vi "Keithley6221Monitor_with_DC.vi"() -> ()   [LabVIEW 2019]
uses:
  Instrument_Setup.vi
  Global/Global Variables/Data_Display_global.vi
  <vilib>/ErrorRing/Error Ring.xnode
  Equipment/Keithley 622x/Keithley 622x.lvlib
  Utility/Monitor Communication/sub-vis/K6221_Check_Queue.vi
  Utility/Monitor Communication/sub-vis/K6221_Open_Queue.vi
  Utility/Monitor Communication/K6221/K6221_Cluster.ctl
  Equipment/Keithley 622x/Configure/Output/Typedefs/KE6221 -- Output Response.ctl
  Equipment/Keithley 622x/Typedefs/KE622x -- On Off Control.ctl
  Equipment/Keithley 622x/Configure/Source/Typedefs/KE622x -- Voltage Limit.ctl
  Equipment/Keithley 622x/Configure/Source/Typedefs/KE622x -- Current Ranges.ctl
  Equipment/Keithley 622x/Configure/Source/Typedefs/KE622x -- Current Range.ctl
panel:
  in  "Current Range In":T1={"Auto Range?"=TRUE, "Man / Selected\nRange"=enum."2nA"}
  in  "Turn Off Output If Voltage Limit? 2":bool=TRUE
  in  "Turn Off Output If Voltage Limit?":bool=TRUE
  in  "Voltage Limit (V)":T3=10.0 min=0.1 max=105.0 step=0.01 format="%.2p"
  in  "Analog Filter State":T4
  in  "Output Response":T5=enum."Slow"
  in  "Combo Box":string(combo)="AC"
  out "Cluster":T6
  # "Set in Instrument Setup!"
  # "K 6221"
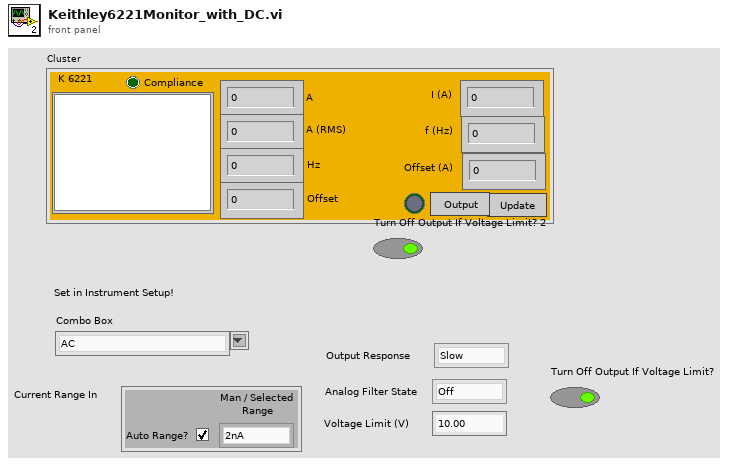
[diagram p1: front panel]
types:
  T1 = typedef "Keithley 622x.lvlib/KE622x -- Current Range.ctl" = cluster{"Auto Range?":bool, "Man / Selected\nRange":T2}
  T2 = typedef "Keithley 622x.lvlib/KE622x -- Current Ranges.ctl" = enum16{"2nA", "20nA", "200nA", "2uA", "20uA", "200uA", "2mA", "20mA", "100mA"}
  T3 = typedef "Keithley 622x.lvlib/KE622x -- Voltage Limit.ctl" = dbl
  T4 = typedef "Keithley 622x.lvlib/KE622x -- On Off Control.ctl" = enum16{"Off", "On"}
  T5 = typedef "Keithley 622x.lvlib/KE6221 -- Output Response.ctl" = enum16{"Fast", "Slow"}
  T6 = typedef "K6221_Cluster.ctl" = cluster{"Plot Window":dbl[][], "A":dbl, "A (RMS)":dbl, "Hz":dbl, "I (A)":dbl, "f (Hz)":dbl, "Update":bool, "Offset":dbl, "Offset (A)":dbl, "Compliance":bool, "Output":bool, "Output Status":bool}
  T7 = typedef "Keithley 622x.lvlib/KE622x -- Current Level.ctl" = dbl
  T8 = typedef "Keithley 622x.lvlib/KE6221 -- Wave Sine Wave Params.ctl" = cluster{"Frequency (Hz)":T9, "Amplitude (A)":T10, "Offset (A)":T7, "Ranging Mode":T11, "Fixed Range":T2, "Playback Mode":T12, "Time (s)":T13, "Num Cycles":T14, "Phase\nMarker?":bool, "Phase Marker (deg)":T15, "Trig Link Line":T16}
  T9 = typedef "Keithley 622x.lvlib/KE6221 -- Wave Frequency.ctl" = dbl
  T10 = typedef "Keithley 622x.lvlib/KE6221 -- Wave Amplitude.ctl" = dbl
  T11 = typedef "Keithley 622x.lvlib/KE6221 -- Wave Ranging Mode.ctl" = enum16{"Best", "Fixed"}
  T12 = typedef "Keithley 622x.lvlib/KE6221 -- Wave Playback Mode.ctl" = enum16{"Time", "Num Cycles"}
  T13 = typedef "Keithley 622x.lvlib/KE6221 -- Wave Playback Time.ctl" = dbl
  T14 = typedef "Keithley 622x.lvlib/KE6221 -- Wave Playback Num Cycles.ctl" = dbl
  T15 = typedef "Keithley 622x.lvlib/KE6221 -- Wave Phase Marker.ctl" = dbl
  T16 = typedef "Keithley 622x.lvlib/KE622x -- Trig Link Line.ctl" = enum16{"1", "2", "3", "4", "5", "6"}
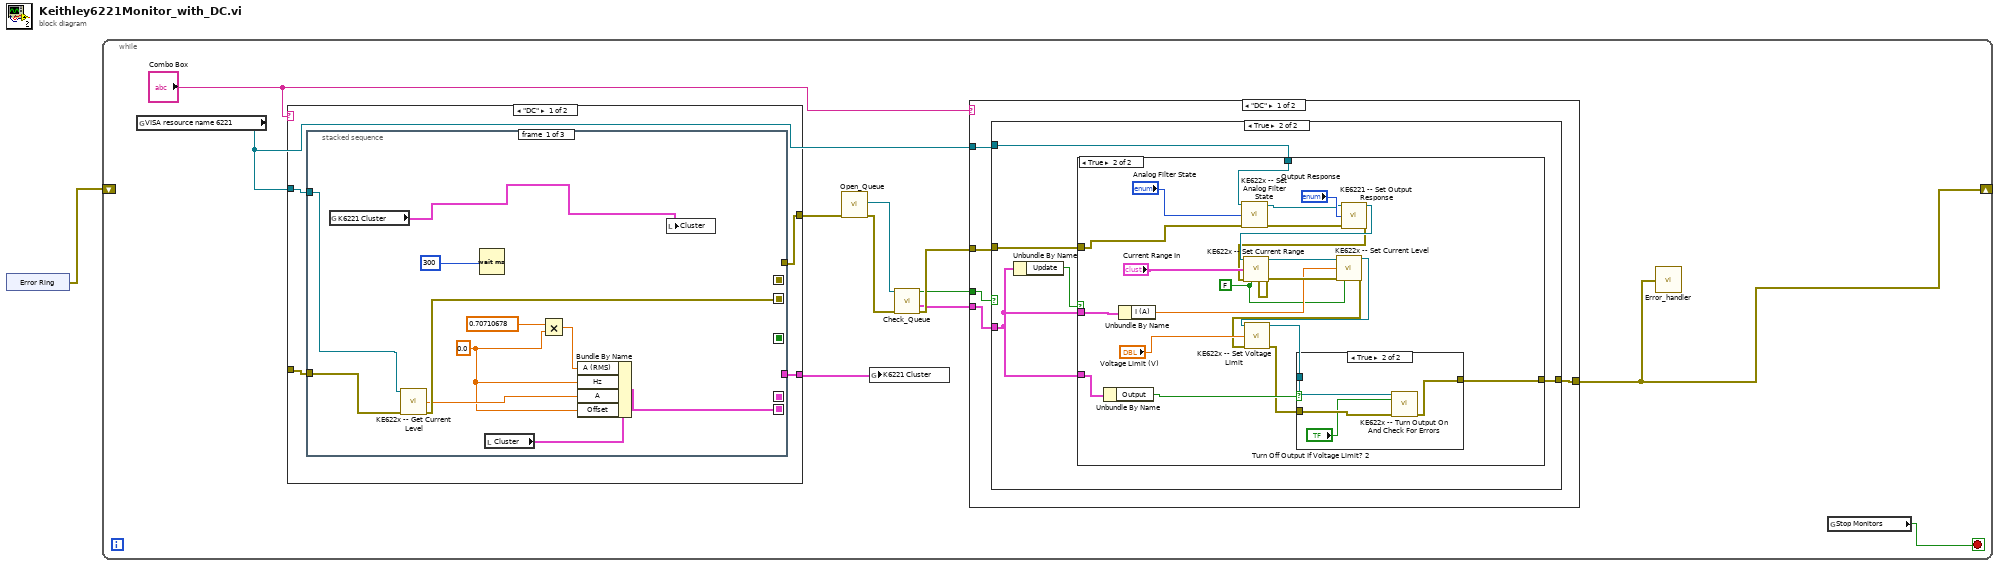
[diagram p0: block diagram]
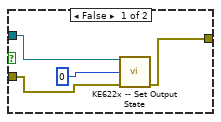
[diagram p4: hidden frame]
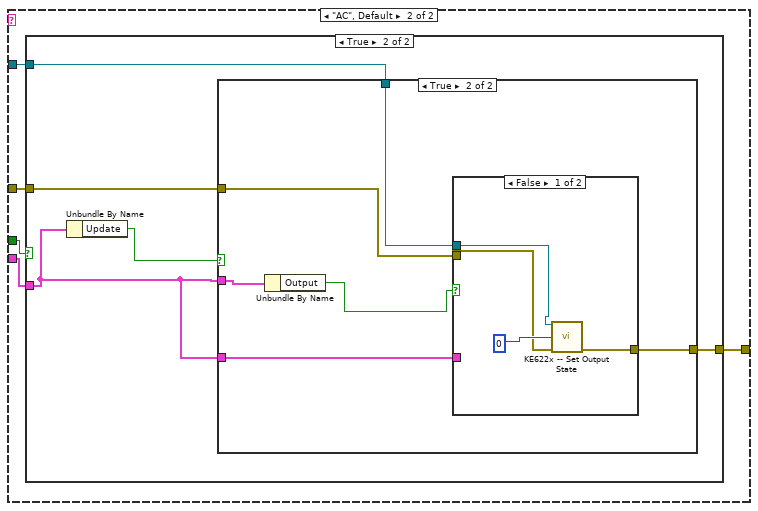
[diagram p5: hidden frame]
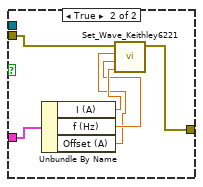
[diagram p8: hidden frame]
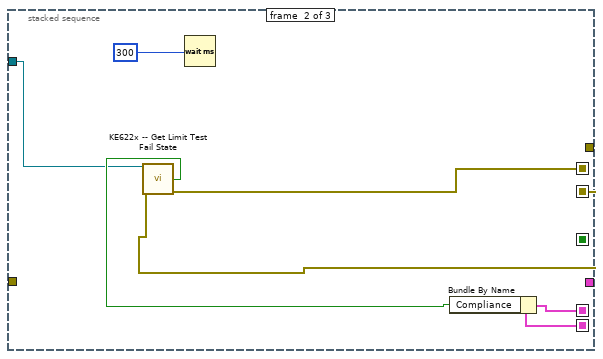
[diagram p9: hidden frame]
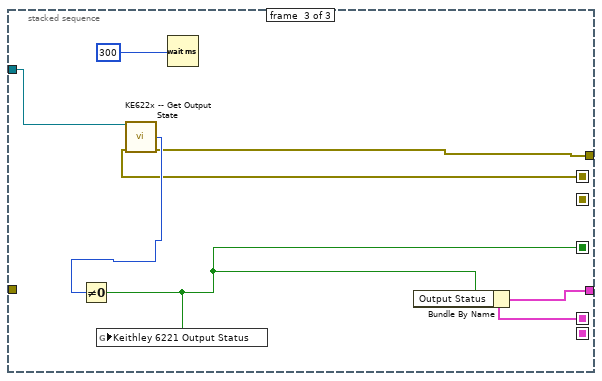
[diagram p10: hidden frame]
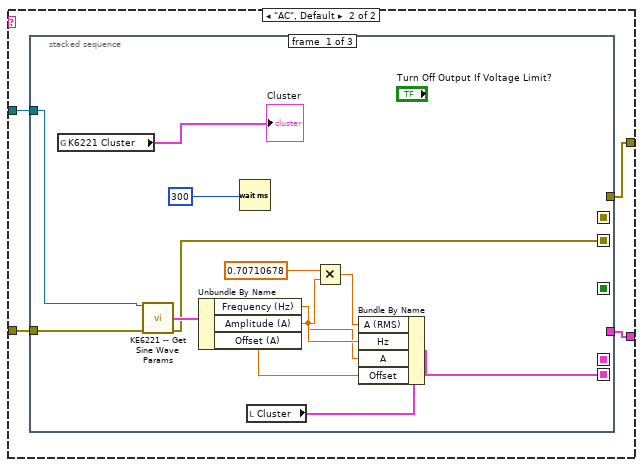
[diagram p11: hidden frame]
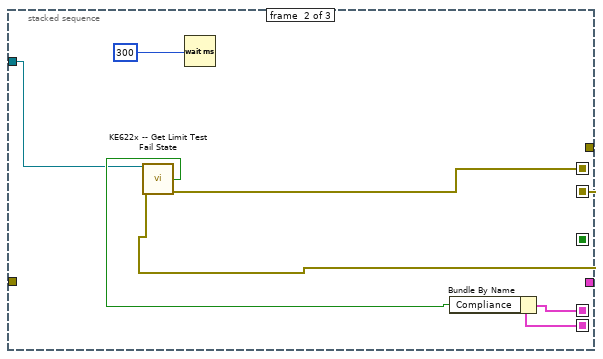
[diagram p12: hidden frame]
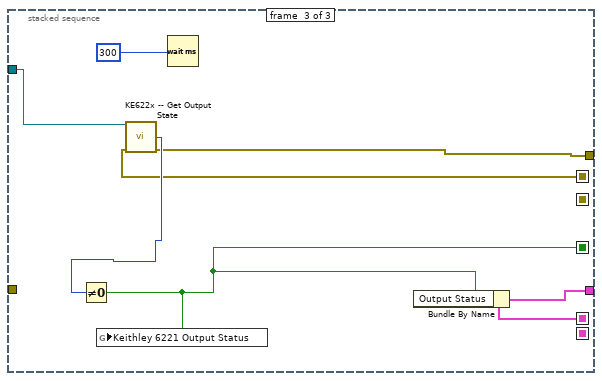
[diagram p13: hidden frame]
diagram:
  n1 = xnode "Error Ring"() -> ("error out"=w1:errorcluster)
  n2 = while {
    shift-right: [w3] -> _
    shift-left: w1 -> [_]
    stop <- w13 stop-if-true
    n3 = global read "Instrument_Setup.vi" "VISA resource name 6221"() -> (w5:refnum<visa-resource-name>)
    n4 = case shown="\"DC\"" "Combo Box" {
      tunnel: [w86 w117] -> w12
      tunnel: [w85 w116] -> w11
      tunnel: w5 -> [w87 w115]
      tunnel: [w84 w114] -> w4
      frame "DC" {
        n5 = stacked-sequence {
          seq-local: [w90 _ _] -> [_ w104 _]
          seq-local: [_ _ w110] -> [_ _ _]
          seq-local: [_ w99 _] -> [_ _ w108]
          seq-local: [w96 _ _] -> [_ w103 _]
          seq-local: [_ w102 _] -> [_ _ w111]
          tunnel: w87 -> [w92 w100 w109]
          tunnel: w86 -> [w91 _ _]
          tunnel: [_ _ w107] -> w85
          tunnel: [_ _ w106] -> w84
          frame #0 {
            w88 = 0.0
            n6 = global read "Data_Display_global.vi" "K6221 Cluster"() -> (w93:T6)
            n7 = call "KE622x -- Get Current Level.vi"("Resource In"=w92, "error in (no error)"=w91) -> ("Current Level (A)"=w89:T7, "error out"=w90:errorcluster)  [unwired: 11 in, 1 out]
            n8 = Wait (ms)(milliseconds to wait=300) -> ()  [unwired: 1 out]
            n9 = local read "Cluster"() -> (w97:T6)
            n10 = Multiply(x=0.70710678, y=w88) -> (x*y=w94:dbl)
            n11 = Bundle By Name(cluster=w97, "A (RMS)"=w94, "Hz"=w88, "A"=w89, "Offset"=w88) -> (w96:T6)
            n12 = local write "Cluster"(w93) -> ()
          }
          frame #1 {
            n13 = call "KE622x -- Get Limit Test Fail State.vi"("Resource In"=w100, "error in (no error)"=w104) -> ("Limit Test Failed (Compliance)?"=w101:bool, "error out"=w99:errorcluster)  [unwired: 11 in, 1 out]
            n14 = Wait (ms)(milliseconds to wait=300) -> ()  [unwired: 1 out]
            n15 = Bundle By Name(cluster=w103, "Compliance"=w101) -> (w102:T6)
          }
          frame #2 {
            n16 = call "KE622x -- Get Output State.vi"("Resource In"=w109, "error in (no error)"=w108) -> ("Output State"=w113:T4, "error out"=w107:errorcluster)  [unwired: 11 in, 1 out]
            n17 = Not Equal To 0?(x=w113) -> (x != 0?=w110:bool)
            n18 = global write "Data_Display_global.vi" "Keithley 6221 Output Status"(w110) -> ()
            n19 = Wait (ms)(milliseconds to wait=300) -> ()  [unwired: 1 out]
            n20 = Bundle By Name(cluster=w111, "Output Status"=w110) -> (w106:T6)
          }
        }
      }
      frame "AC", Default {
        n21 = stacked-sequence {
          seq-local: [w128 _ _] -> [_ w136 _]
          seq-local: [_ _ w142] -> [_ _ _]
          seq-local: [_ w131 _] -> [_ _ w140]
          seq-local: [w121 _ _] -> [_ w135 _]
          seq-local: [_ w134 _] -> [_ _ w143]
          tunnel: w115 -> [w124 w132 w141]
          tunnel: w117 -> [w123 _ _]
          tunnel: [_ _ w139] -> w116
          tunnel: [_ _ w138] -> w114
          frame #0 {
            n22 = global read "Data_Display_global.vi" "K6221 Cluster"() -> (→"Cluster":T6)
            n23 = call "KE6221 -- Get Sine Wave Params.vi"("Resource In"=w124, "error in (no error)"=w123) -> ("Sine Wave Params"=w130:T8, "error out"=w128:errorcluster)  [unwired: 11 in, 1 out]
            n24 = Unbundle By Name(w130) -> ("Frequency (Hz)"=w126:T9, "Amplitude (A)"=w120:T10, "Offset (A)"=w125:T7)
            n25 = Wait (ms)(milliseconds to wait=300) -> ()  [unwired: 1 out]
            n26 = local read "Cluster"() -> (w127:T6)
            n27 = Multiply(x=0.70710678, y=w120) -> (x*y=w118:T10)
            n28 = Bundle By Name(cluster=w127, "A (RMS)"=w118, "Hz"=w126, "A"=w120, "Offset"=w125) -> (w121:T6)
          }
          frame #1 {
            n29 = call "KE622x -- Get Limit Test Fail State.vi"("Resource In"=w132, "error in (no error)"=w136) -> ("Limit Test Failed (Compliance)?"=w133:bool, "error out"=w131:errorcluster)  [unwired: 11 in, 1 out]
            n30 = Wait (ms)(milliseconds to wait=300) -> ()  [unwired: 1 out]
            n31 = Bundle By Name(cluster=w135, "Compliance"=w133) -> (w134:T6)
          }
          frame #2 {
            n32 = call "KE622x -- Get Output State.vi"("Resource In"=w141, "error in (no error)"=w140) -> ("Output State"=w145:T4, "error out"=w139:errorcluster)  [unwired: 11 in, 1 out]
            n33 = Not Equal To 0?(x=w145) -> (x != 0?=w142:bool)
            n34 = global write "Data_Display_global.vi" "Keithley 6221 Output Status"(w142) -> ()
            n35 = Wait (ms)(milliseconds to wait=300) -> ()  [unwired: 1 out]
            n36 = Bundle By Name(cluster=w143, "Output Status"=w142) -> (w138:T6)
          }
        }
      }
    }
    n37 = call-poly "Open_Queue.vi"("error in (no error)"=w11) -> ("error out"=w10:errorcluster, "queue out"=w9:refnum<queue>)  [unwired: 9 in]
    n38 = global write "Data_Display_global.vi" "K6221 Cluster"(w4) -> ()
    n39 = call-poly "Check_Queue.vi"("error in (no error)"=w10, "queue"=w9) -> ("error out"=w8:errorcluster, "Command (in)"=w7:T6, "New Entries?"=w6:bool)  [unwired: 6 in]
    n40 = case shown="\"DC\"" "Combo Box" {
      tunnel: w8 -> [w16 w60]
      tunnel: w7 -> [w17 w59]
      tunnel: w6 -> [w18 w58]
      tunnel: w5 -> [w15 w57]
      tunnel: [w14 w56] -> w3
      frame "DC" {
        n41 = case shown="True" w18 {
          tunnel: w16 -> [w19 w22]
          tunnel: w17 -> [_ w21]
          tunnel: w15 -> [_ w23]
          tunnel: [w19 w20] -> w14
          frame False {
          }
          frame True {
            n42 = Unbundle By Name(w21) -> ("Update"=w24:bool)
            n43 = case shown="True" w24 {
              tunnel: w23 -> [_ w44]
              tunnel: w22 -> [w25 w45]
              tunnel: w21 -> [_ w47]
              tunnel: w21 -> [_ w46]
              tunnel: [w25 w26] -> w20
              frame False {
              }
              frame True {
                w33 = FALSE ("Read Back Set Values? (T)")
                n44 = Unbundle By Name(w47) -> ("Output"=w29:bool)
                n45 = Unbundle By Name(w46) -> ("I (A)"=w35:dbl)
                n46 = call "KE622x -- Set Analog Filter State.vi"("Resource In"=w44, "Analog Filter State"="Analog Filter State", "error in (no error)"=w45) -> ("Resource Out (dupl)"=w41:refnum<visa-resource-name>, "error out"=w40:errorcluster)  [unwired: 11 in]
                n47 = call "KE6221 -- Set Output Response.vi"("Resource In"=w41, "KE6221 Output Response"="Output Response", "error in (no error)"=w40) -> ("Resource Out (dupl)"=w39:refnum<visa-resource-name>, "error out"=w37:errorcluster)  [unwired: 11 in]
                n48 = call "KE622x -- Set Current Range.vi"("Resource In"=w39, "Current Range In"="Current Range In", "error in (no error)"=w37, "Read Back Set Values? (T)"=w33) -> ("Resource Out (dupl)"=w34:refnum<visa-resource-name>, "error out"=w36:errorcluster)  [unwired: 9 in, 1 out]
                n49 = call "KE622x -- Set Current Level.vi"("Resource In"=w34, "Current Level (A) In"=w35, "error in (no error)"=w36, "Read Back Set Value? (T)"=w33) -> ("Resource Out (dupl)"=w31:refnum<visa-resource-name>, "error out"=w30:errorcluster)  [unwired: 9 in, 1 out]
                n50 = call "KE622x -- Set Voltage Limit.vi"("Resource In"=w31, "Voltage Limit (V)"="Voltage Limit (V)", "error in (no error)"=w30) -> ("Resource Out (dupl)"=w28:refnum<visa-resource-name>, "error out"=w27:errorcluster)  [unwired: 11 in]
                n51 = case shown="True" w29 {
                  tunnel: w28 -> [w48 w55]
                  tunnel: w27 -> [w50 w54]
                  tunnel: [w49 w53] -> w26
                  frame False {
                    n52 = call "KE622x -- Set Output State.vi"("Resource In"=w48, "Output State"=0, "error in (no error)"=w50) -> ("error out"=w49:errorcluster)  [unwired: 11 in, 1 out]
                  }
                  frame True {
                    n53 = call "KE622x -- Turn Output On And Check For Errors.vi"("Resource In"=w55, "Turn Off Output If Compliance?"="Turn Off Output If Voltage Limit? 2", "error in (no error)"=w54) -> ("error out"=w53:errorcluster)  [unwired: 9 in, 3 out]
                  }
                }
              }
            }
          }
        }
      }
      frame "AC", Default {
        n54 = case shown="True" w58 {
          tunnel: w60 -> [w61 w64]
          tunnel: w59 -> [_ w63]
          tunnel: w57 -> [_ w65]
          tunnel: [w61 w62] -> w56
          frame False {
          }
          frame True {
            n55 = Unbundle By Name(w63) -> ("Update"=w66:bool)
            n56 = case shown="True" w66 {
              tunnel: w65 -> [_ w73]
              tunnel: w64 -> [w67 w72]
              tunnel: w63 -> [_ w71]
              tunnel: w63 -> [_ w70]
              tunnel: [w67 w69] -> w62
              frame False {
              }
              frame True {
                n57 = Unbundle By Name(w71) -> ("Output"=w68:bool)
                n58 = case shown="False" w68 {
                  tunnel: w73 -> [w76 _]
                  tunnel: w72 -> [w75 w83]
                  tunnel: [w74 w82] -> w69
                  tunnel: w70 -> [_ w81]
                  frame False {
                    n59 = call "KE622x -- Set Output State.vi"("Resource In"=w76, "Output State"=0, "error in (no error)"=w75) -> ("error out"=w74:errorcluster)  [unwired: 11 in, 1 out]
                  }
                  frame True {
                    n60 = Unbundle By Name(w81) -> ("I (A)"=w80:dbl, "f (Hz)"=w79:dbl, "Offset (A)"=w78:dbl)
                    n61 = call "Set_Wave_Keithley6221.vi"("I (A)"=w80, "f (Hz)"=w79, "Offset (A)"=w78, "Error in"=w83) -> ("Erro out"=w82:errorcluster)  [unwired: 5 in]
                  }
                }
              }
            }
          }
        }
      }
    }
    n62 = call "Error_handler.vi"("error constant"=w3) -> ()
    n63 = global read "Data_Display_global.vi" "Stop Monitors"() -> (w13:bool)
  }
